vi "Handle UI events.vi"(8 "error in (no error)":errorcluster, 10 "Control in":refnum<vi>, 11 "DatagridElement in":refnum<class "DatagridElement.lvclass">) -> (0 "error out":errorcluster, 2 "Tabbed out?":bool, 3 "DatagridElement out":refnum<class "DatagridElement.lvclass">)   [LabVIEW 2018, in "D Datagrid Library.lvlib" / "DatagridElement.lvclass"]
doc: "Handles mousedown, keyboard, and other events. Override this VI if you want additional functionality for a specific element type."
uses:
  DatagridElement.lvclass
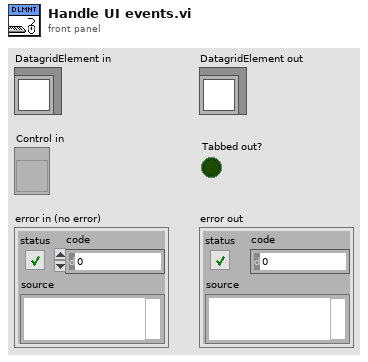
[diagram p1: front panel]
types:
  T1 = typedef "eventvkey.ctl" = enum16{"ASCII", "Enter", "Return", "Shift", "Ctrl", "Alt", "Cmd", "Opt", "Caps", "NumLock", "Clear", "Break", "Up", "Down", "Left", "Right", "Insert", "Delete", "Home", "End", "PageUp", "PageDown", "Escape", "Help", "Pause", "ScrollLock", "F1", "F2", "F3", "F4", "F5", "F6", "F7", "F8", "F9", "F10", "F11", "F12", "F13", "F14", "F15", "F16", "F17", "F18", "F19", "F20", "F21", "F22", "F23", "F24", "Play", "VolumeUp", "VolumeDown", "Mute", "Two Byte Char"}
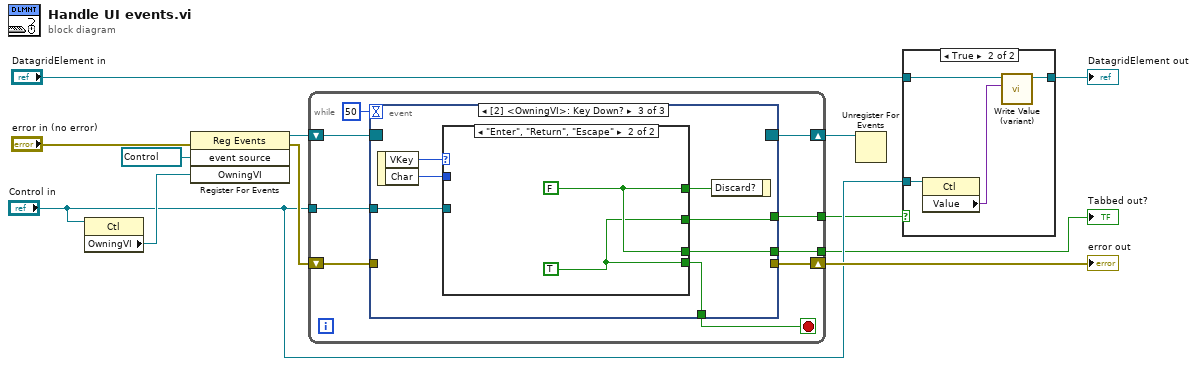
[diagram p0: block diagram]
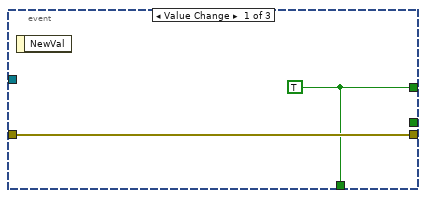
[diagram p3: hidden frame]
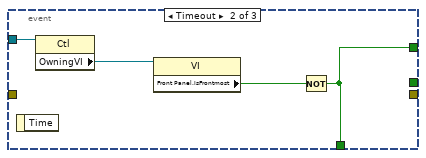
[diagram p4: hidden frame]
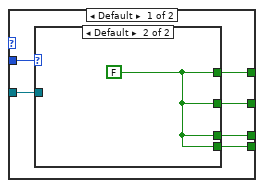
[diagram p5: hidden frame]
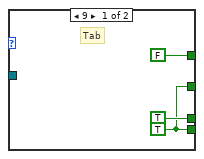
[diagram p6: hidden frame]
diagram:
  n1 = property class="Ctl"(reference="Control in") -> ("OwningVI"=w8:refnum<vi>)  [unwired: 1 in, 2 out]
  n2 = register-events(error in="error in (no error)", refnum<vi> refnum ("event source"), w8) -> (reference out=w10:refnum<event-registration>, error out=w11:errorcluster)  [unwired: 1 in]
  n3 = while {
    shift-right: [w20] -> w9
    shift-left: w10 -> [w21]
    shift-right: [w19] -> w7
    shift-left: w11 -> [w18]
    tunnel: "Control in" -> [w15]
    tunnel: [w14] -> w4
    tunnel: [w13] -> w3
    stop <- w17 stop-if-true
    n4 = event shown="[2] <OwningVI>: Key Down?" {
      selector: w21 -> [_ _ _]
      dyn-events: [_ _ _] -> w20
      timeout: 50 -> [_ _ _]
      tunnel: [w23 _ _] -> w19
      tunnel: w18 -> [w23 _ _]
      tunnel: [w22 w24 w33] -> w17
      tunnel: w15 -> [_ w27 w29]
      tunnel: [_ _ w30] -> w14
      tunnel: [w22 w24 w28] -> w13
      event Value Change {
        w22 = TRUE
        n5 = event-data() -> ()  [unwired: 1 in, 1 out]
      }
      event Timeout {
        n6 = event-data() -> ()  [unwired: 1 in, 1 out]
        n7 = property class="Ctl"(reference=w27) -> ("OwningVI"=w26:refnum<vi>)  [unwired: 1 in, 2 out]
        n8 = property class="VI"(reference=w26) -> ("Front Panel.IsFrontmost"=w25:bool)  [unwired: 1 in, 2 out]
        n9 = Not(x=w25) -> (.not. x?=w24:bool)
      }
      event Key Down? {
        n10 = event-data() -> ("VKey"=w34:T1, "Char"=w31:i16)  [unwired: 1 in]
        n11 = case shown="\"Enter\", \"Return\", \"Escape\"" w34 {
          tunnel: [w38 w45] -> w33
          tunnel: [w40 w46] -> w32
          tunnel: w31 -> [w39 _]
          tunnel: [w37 w46] -> w30
          tunnel: w29 -> [w36 _]
          tunnel: [w35 w45] -> w28
          frame Default {
            n12 = case shown="Default" w39 {
              tunnel: [FALSE ("Discard?") w44] -> w40
              tunnel: [w41 w44] -> w38
              tunnel: [TRUE ("Discard?") w44] -> w37
              tunnel: w36 -> [_ _]
              tunnel: [w41 w44] -> w35
              frame 9 {
                w41 = TRUE ("Discard?")
                # "Tab"
              }
              frame Default {
                w44 = FALSE ("Discard?")
              }
            }
          }
          frame "Enter", "Return", "Escape" {
            w46 = FALSE ("Discard?")
            w45 = TRUE ("x = y?")
          }
        }
        n13 = event-data("Discard?"=w32) -> ()  [unwired: 1 in, 1 out]
      }
    }
  }
  "error out" <- w7
  "Tabbed out?" <- w4
  n14 = Unregister For Events(event registration refnum=w9) -> ()  [unwired: 1 in, 1 out]
  n15 = case shown="True" w3 {
    tunnel: "DatagridElement in" -> [w47 w51]
    tunnel: [w47 w50] -> w6
    tunnel: "Control in" -> [_ w48]
    frame False {
    }
    frame True {
      n16 = property class="Ctl"(reference=w48) -> ("Value"=w49:variant)  [unwired: 1 in, 2 out]
      n17 = call-dynamic "Write Value (variant).vi"("Variant"=w49, "DatagridElement in"=w51) -> ("DatagridElement out"=w50:refnum<class "DatagridElement.lvclass">)  [unwired: 8 in, 1 out]
    }
  }
  "DatagridElement out" <- w6
